vi "GlobalVariables.vi"() -> ()   [LabVIEW 2018]
panel:
  out "HistogramEnabled":bool
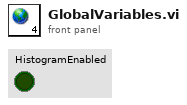
[diagram p1: front panel]
diagram:
